vi "GA Cmp Buf Sts.vi"(8 "error in (no error)":errorcluster caption="错误输入（无错误）", 10 "pCount":u16, 11 "pStatus":i16) -> (0 "error out":errorcluster caption="错误输出", 1 "function return":i32, 2 "pCount out":u16, 3 "pStatus out":i16)   [LabVIEW 2015, in "GAS.lvlib"]
doc: "extern \"C\" __declspec(dllimport) int GA_CmpBufSts(short *pStatus,unsigned short *pCount);"
uses:
  <userlib>/BP_GAS/GAS.lvlib
  <userlib>/BP_GAS/GAS.dll
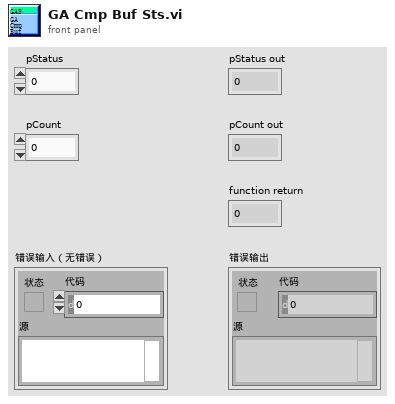
[diagram p1: front panel]
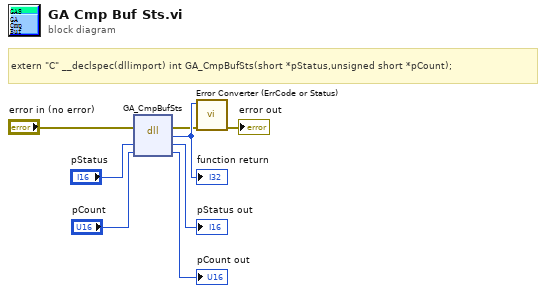
[diagram p0: block diagram]
diagram:
  # "extern \"C\" __declspec(dllimport) int GA_CmpBufSts(short *pStatus,unsigned short *pCount);"
  n1 = dll-call lib="E:/Program Files (x86)/National Instruments/LabVIEW 2015/user.lib/BP_GAS/GAS.*" fn="GA_CmpBufSts"(error in="error in (no error)", "pStatus"="pStatus", "pCount"="pCount") -> (error out=w2:errorcluster, w8:i32, "pStatus"=→"pStatus out":i16, "pCount"=→"pCount out":u16)  [unwired: 2 in, 1 out]
  "function return" <- w8
  n2 = call "Error Converter (ErrCode or Status).vi"("error in (no error)"=w2, "error code"=w8) -> ("error out"=→"error out":errorcluster)  [unwired: 9 in]
